vi "Measurement.vi"(8 "error in (no error)":errorcluster, 11 "YP03-60_Y in":refnum<class "YP03-60_Y.lvclass">) -> (0 "error out":errorcluster, 2 "Output":dbl[](array[numeric]), 3 "YP03-60_Y out":refnum<class "YP03-60_Y.lvclass">)   [LabVIEW 2020, in "PowerControl.lvlib" / "YP03-60_Y.lvclass"]
uses:
  YP03-60_Y.lvclass
  YP03-60_X/YP03-60_X.lvclass
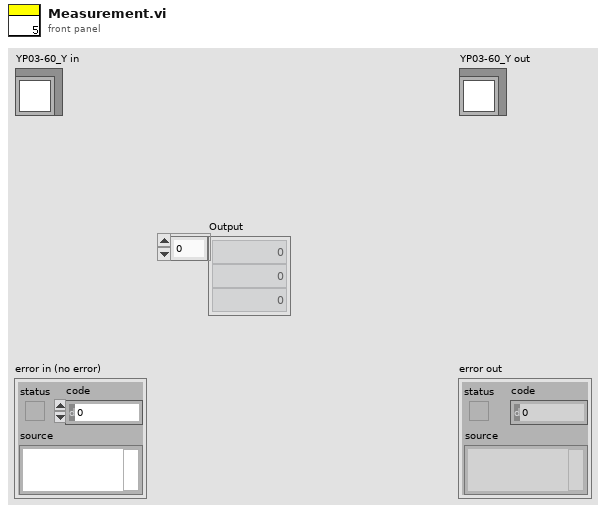
[diagram p1: front panel]
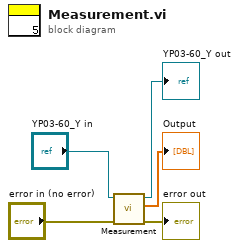
[diagram p0: block diagram]
diagram:
  n1 = call-parent "Measurement.vi"("error in (no error)"="error in (no error)", "YP03-60_X in"="YP03-60_Y in") -> ("error out"=→"error out":errorcluster, "Output"=→"Output":dbl[], "YP03-60_X out"=→"YP03-60_Y out":refnum<class "YP03-60_Y.lvclass">)  [unwired: 7 in]
